vi "Master Controller_Create.vi"(0 "reference in":refnum<class "Master Controller.lvclass">, 5 "error in (no error)":errorcluster) -> (14 "reference out":refnum<class "Master Controller.lvclass">, 19 "error out":errorcluster)   [LabVIEW 2016, in "Master Controller.lvclass"]
doc: "Constructor."
uses:
  Master Controller.lvclass
  C:/Program Files (x86)/National Instruments/LabVIEW 2016/vi.lib/addons/_AddQ/G#Object/G#Object.lvclass
  <vilib>/addons/_AddQ/G#Object/G#Object.lvclass
  File Controller_llb/File Controller.lvclass
  Devices Controller_llb/Devices Controller.lvclass
  Items Controller_llb/Items Controller.lvclass
  GUI/GUI Controller_llb/GUI Controller.lvclass
  Notification Controller_class/Notification Controller.lvclass
  PartsTracking Controller_class/PartsTracking Controller.lvclass
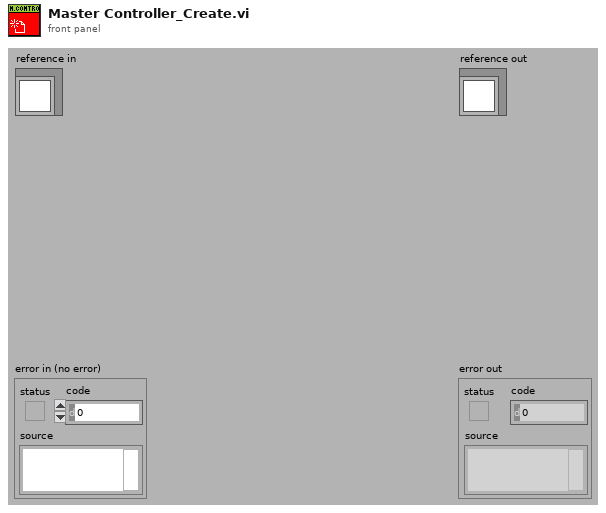
[diagram p1: front panel]
types:
  T1 = typedef "Master Controller.lvclass/ObjectAttributesRef.ctl" = refnum<data-value>
  T2 = typedef "Master Controller.lvclass/ClassAttributesRef.ctl" = refnum<data-value>
  T3 = typedef "Master Controller.lvclass/ClassAttributes.ctl" = cluster{"Dummy":bool, "Master Controller_ref":refnum<class "Master Controller.lvclass">}
  T4 = typedef "Master Controller.lvclass/ObjectAttributes.ctl" = cluster{"MyAttribute":dbl, "Devices Controller_ref":refnum<class "Devices Controller.lvclass">, "File Controller_ref":refnum<class "File Controller.lvclass">, "Items Controller_ref":refnum<class "Items Controller.lvclass">, "GUI Controller_ref":refnum<class "GUI Controller.lvclass">, "NotificationController_ref":refnum<class "Notification Controller.lvclass">, "PartsTracking Controller_ref":refnum<class "PartsTracking Controller.lvclass">}
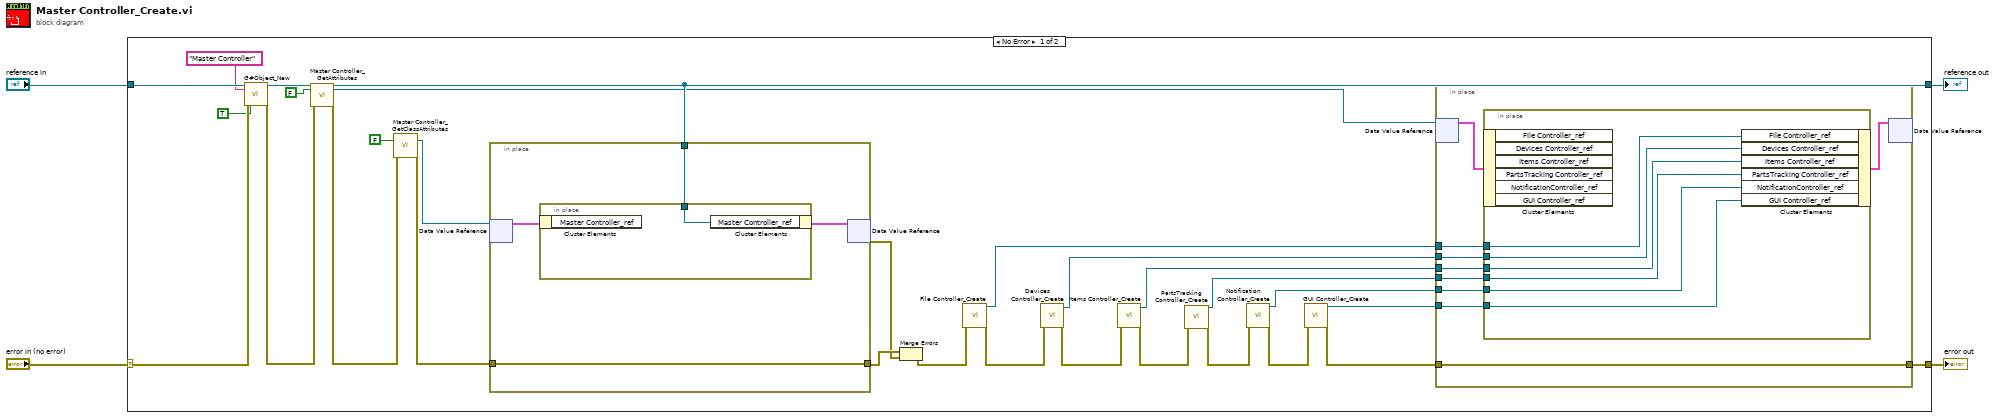
[diagram p0: block diagram]
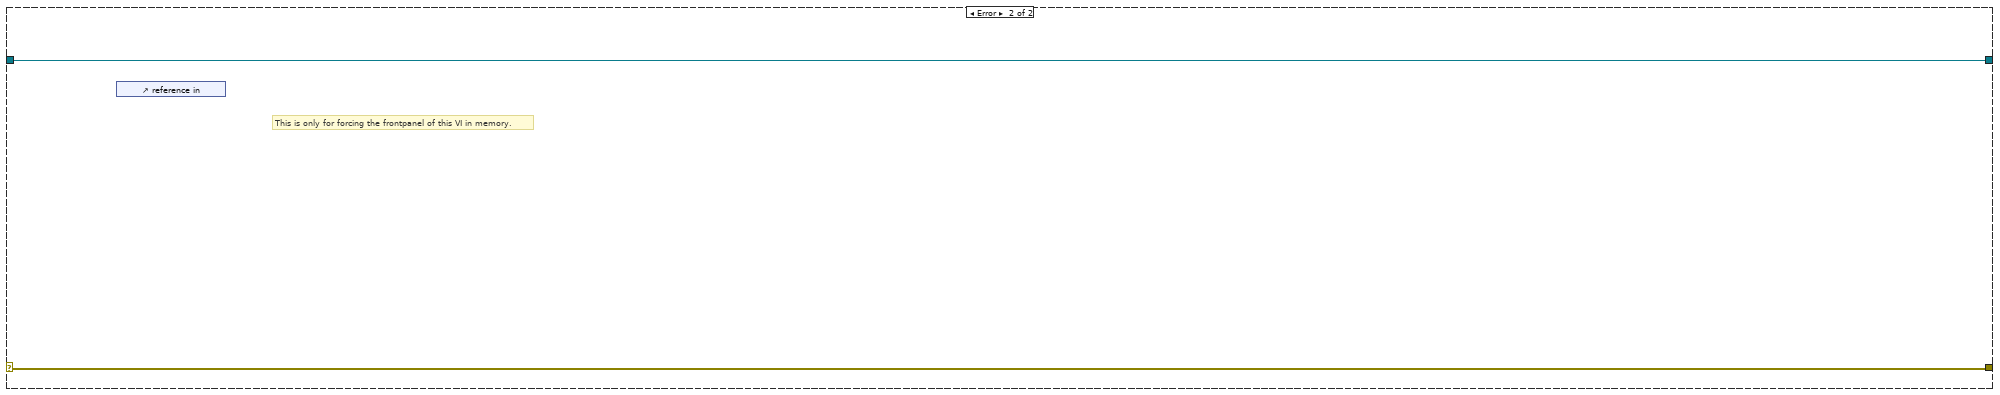
[diagram p2: hidden frame]
diagram:
  n1 = case shown="No Error" "error in (no error)" {
    selector: "error in (no error)" -> [w32 w55]
    tunnel: [w18 w55] -> w3
    tunnel: [w22 w54] -> w1
    tunnel: "reference in" -> [w33 w54]
    frame No Error {
      n2 = call <vilib>:"G#Object_New.vi"("reference in"=w33, "object name"="Master Controller", "error in (no error)"=w32, "user counter (T)?"=TRUE ("User Counter")) -> ("reference out"=w28:refnum<class "Master Controller.lvclass">, "error out"=w27:errorcluster)  [unwired: 13 in, 1 out]
      n3 = call "Master Controller_GetAttributes.vi"("reference in"=w28, "return data? (T)"=FALSE ("return data"), "error in (no error)"=w27) -> ("reference out"=w22:refnum<class "Master Controller.lvclass">, "attributes ref"=w17:T1, "error out"=w25:errorcluster)  [unwired: 13 in, 1 out]
      n4 = call "Master Controller_GetClassAttributes.vi"("return data? (T)"=FALSE, "error in (no error)"=w25) -> ("class attributes ref"=w23:T2, "error out"=w24:errorcluster)  [unwired: 14 in, 2 out]
      n5 = in-place {
        in-place-border: w24 -> [w50]
        in-place-border: [w50] -> w30
        in-place-border: w22 -> [w49]
        n6 = in-place-dvr #1(w23) -> (w51:T3)  [unwired: 1 out]
        n7 = in-place {
          in-place-border: w49 -> [w53]
          n8 = in-place-cluster #2(w51) -> ()  [unwired: 1 out]
          n9 = in-place-cluster #2("Master Controller_ref"=w53) -> (w52:T3)
        }
        n10 = in-place-dvr #1(w52) -> (w29:errorcluster)  [unwired: 1 out]
      }
      n11 = Merge Errors(w30, w29) -> (w19:errorcluster)
      n12 = call "File Controller_Create.vi"("error in (no error)"=w19) -> ("reference out"=w13:refnum<class "File Controller.lvclass">, "error out"=w16:errorcluster)  [unwired: 17 in]
      n13 = call "Devices Controller_Create.vi"("error in (no error)"=w16) -> ("error out"=w15:errorcluster, "reference out"=w12:refnum<class "Devices Controller.lvclass">)  [unwired: 9 in]
      n14 = call "Items Controller_Create.vi"("error in (no error)"=w15) -> ("error out"=w6:errorcluster, "reference out"=w11:refnum<class "Items Controller.lvclass">)  [unwired: 9 in]
      n15 = call "PartsTracking Controller_Create.vi"("error in (no error)"=w6) -> ("reference out"=w7:refnum<class "PartsTracking Controller.lvclass">, "error out"=w5:errorcluster)  [unwired: 17 in]
      n16 = call "Notification Controller_Create.vi"("error in (no error)"=w5) -> ("reference out"=w8:refnum<class "Notification Controller.lvclass">, "error out"=w9:errorcluster)  [unwired: 17 in]
      n17 = call "GUI Controller_Create.vi"("error in (no error)"=w9) -> ("reference out"=w10:refnum<class "GUI Controller.lvclass">, "error out"=w14:errorcluster)  [unwired: 17 in]
      n18 = in-place {
        in-place-border: w14 -> [w40]
        in-place-border: [w40] -> w18
        in-place-border: w13 -> [w39]
        in-place-border: w12 -> [w38]
        in-place-border: w11 -> [w37]
        in-place-border: w7 -> [w36]
        in-place-border: w10 -> [w35]
        in-place-border: w8 -> [w34]
        n19 = in-place-dvr #3(w17) -> (w41:T4)  [unwired: 1 out]
        n20 = in-place {
          in-place-border: w39 -> [w48]
          in-place-border: w38 -> [w47]
          in-place-border: w37 -> [w46]
          in-place-border: w36 -> [w45]
          in-place-border: w35 -> [w44]
          in-place-border: w34 -> [w43]
          n21 = in-place-cluster #4(w41) -> ()  [unwired: 6 out]
          n22 = in-place-cluster #4("File Controller_ref"=w48, "Devices Controller_ref"=w47, "Items Controller_ref"=w46, "PartsTracking Controller_ref"=w45, "NotificationController_ref"=w43, "GUI Controller_ref"=w44) -> (w42:T4)
        }
        n23 = in-place-dvr #3(w42) -> ()  [unwired: 2 out]
      }
    }
    frame Error {
      # "This is only for forcing the frontpanel of this VI in memory."
      n24 = control-ref of="reference in"() -> ()  [unwired: 1 out]
    }
  }
  "error out" <- w3
  "reference out" <- w1
